vi "2_1.vi"() -> ()   [LabVIEW 2010]
panel:
  out "x+y":dbl
  out "Waveform Chart":dbl(graph)
  in  "stop":bool
  in  "õ":dbl
  in  "ó":dbl
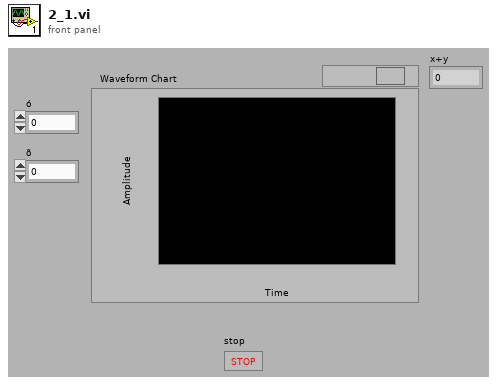
[diagram p1: front panel]
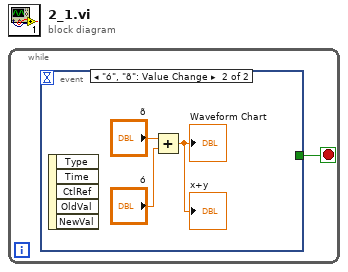
[diagram p0: block diagram]
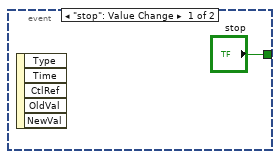
[diagram p2: hidden frame]
diagram:
  n1 = while {
    stop <- w1 stop-if-true
    n2 = event shown="[1] \"ó\", \"õ\": Value Change" {
      selector: _ -> [_ _]
      dyn-events: _ -> [_ _]
      timeout: _ -> [_ _]
      tunnel: ["stop" _] -> w1
      event "stop": Value Change {
        n3 = event-data() -> ()  [unwired: 1 in, 5 out]
      }
      event "ó", "õ": Value Change {
        n4 = event-data() -> ()  [unwired: 1 in, 5 out]
        n5 = Add(x="õ", y="ó") -> (x+y=→"Waveform Chart" →"x+y":dbl)
      }
    }
  }
